vi "Separator_Single_Frame_Displ-3.vi"(3 "error IN":errorcluster, 4 "[IN] Dot matrix with \nstatuses for potentially \nmoving dots":i16[][](array[numeric]), 5 "[IN] Possibly\nMoving (X,Y)":dbl[][](array[numeric]), 6 "[IN] Single Displ":dbl[][](array[numeric])) -> (0 "error OUT":errorcluster, 1 "[OUT] Dot matrix with \nstatuses for potentially \nmoving dots":i16[][](array[numeric]), 2 "[OUT] Single Displ\nw/t problems":dbl[][](array[numeric]))   [LabVIEW 2017]
panel:
  out "Numeric\nof \"+1\" \nevents":i32
  out "2dots to 1dot":dbl[][](array[numeric])
  out "1dot to 2dots":dbl[][](array[numeric])
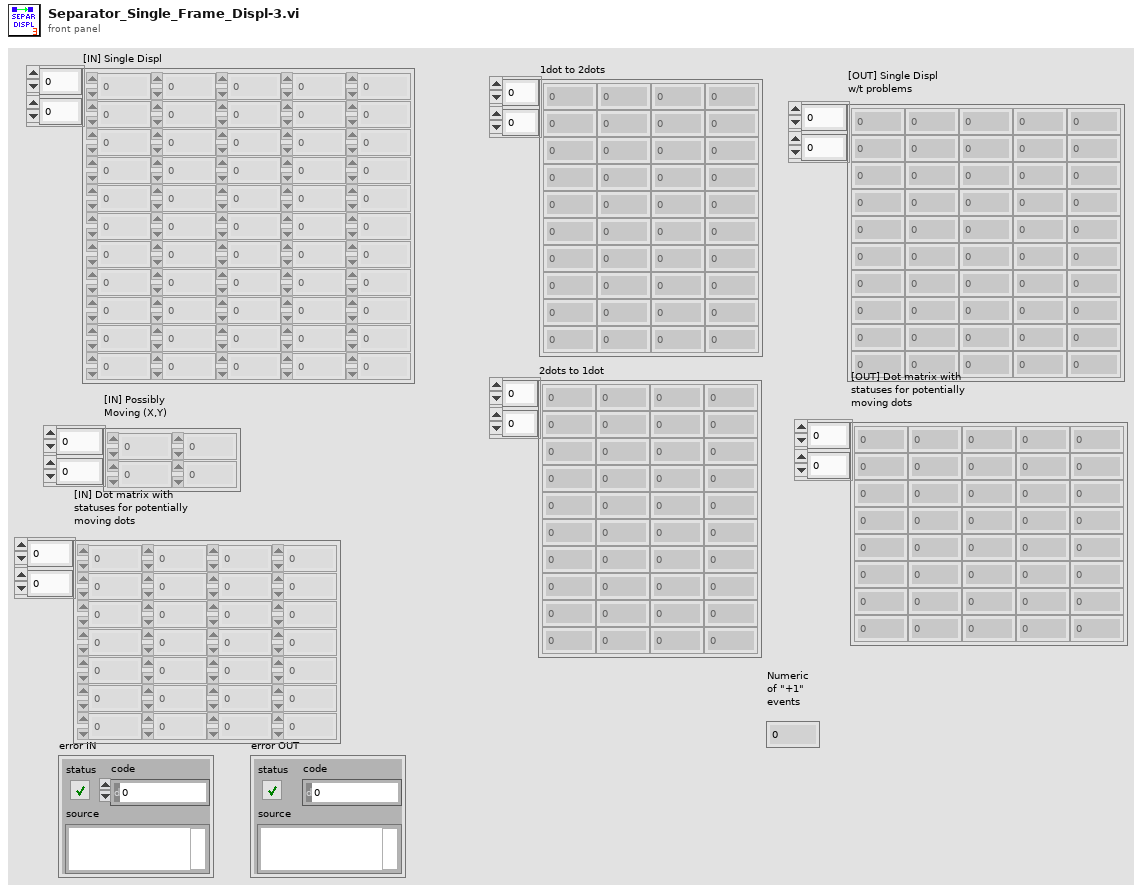
[diagram p1: front panel]
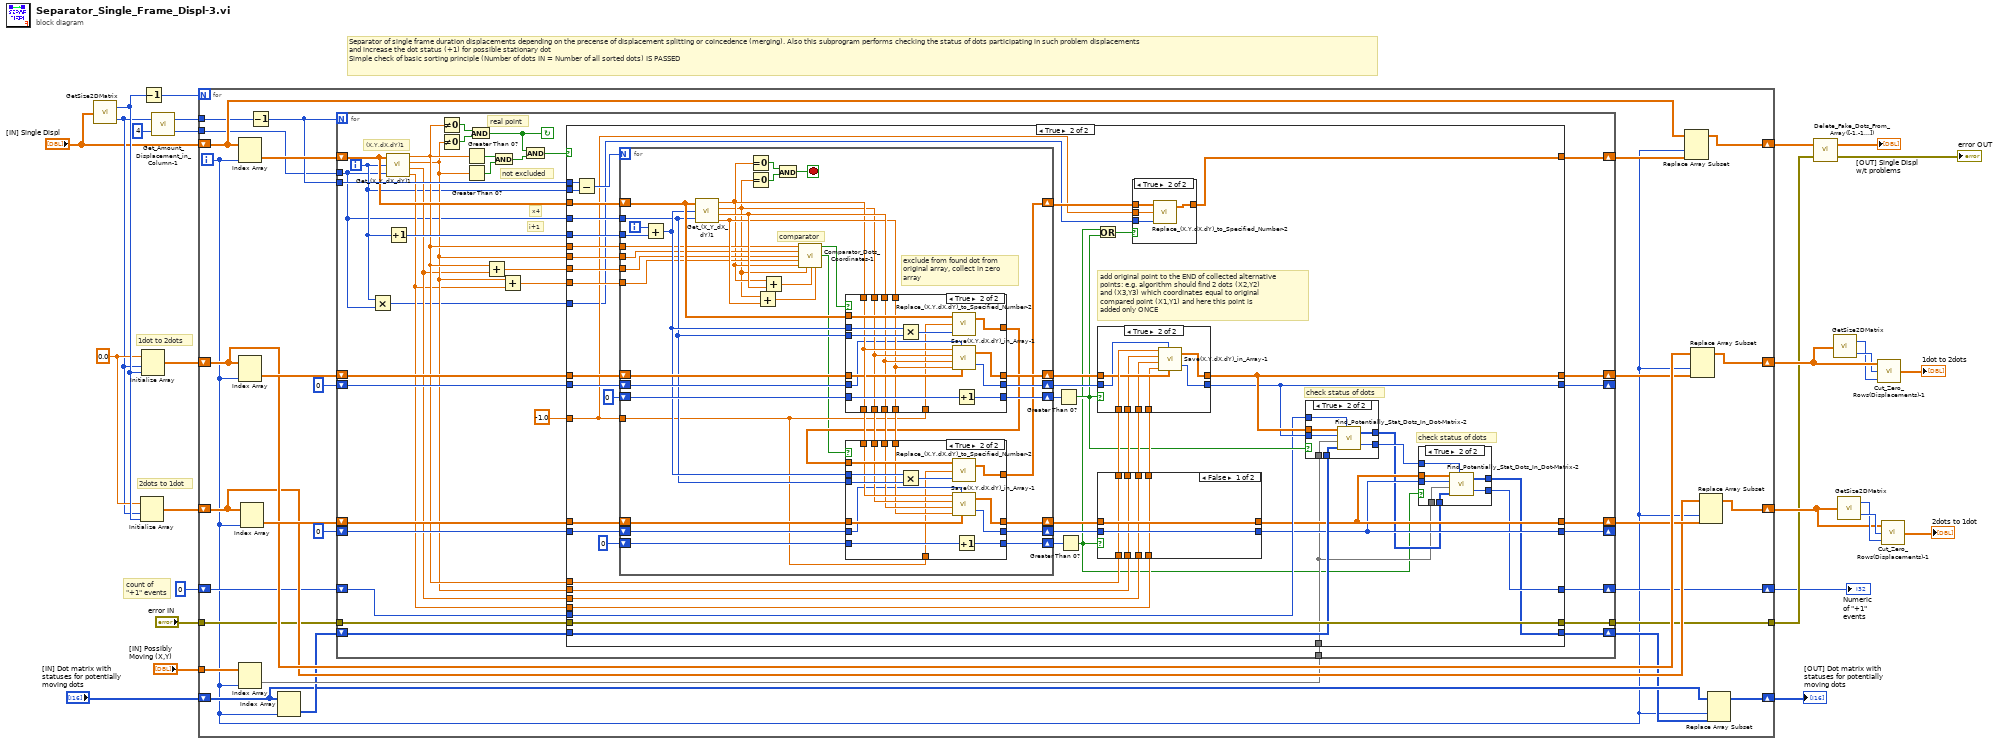
[diagram p0: block diagram]
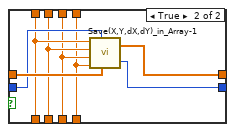
[diagram p6: hidden frame]
diagram:
  w18 = 0.0 ("element")
  # "count of \n\"+1\" events"
  # "2dots to 1dot"
  # "1dot to 2dots"
  # "Separator of single frame duration displacements depending on the precense of displacement splitting or coincedence (merging). Also this subprogram performs checking the status of dots participating in such problem displacements\nand increase the dot status (+1) for possible stationary dot \nSimple check of basic sorting principle (Number of dots IN = Number of all sorted dots) IS PASSED"
  n1 = call "GetSize2DMatrix.vi"("Array IN (2D)"="[IN] Single Displ") -> ("# Cols"=w19:i32, "# Rows"=w13:i32)
  n2 = Initialize Array(w18, w13, w19) -> (w26:dbl[][])
  n3 = Initialize Array(w18, w13, w19) -> (w27:dbl[][])
  n4 = Decrement(x=w19) -> (x-1=w28:i32)
  n5 = call "Get_Amount_Displacement_in_Column-1.vi"("multiplier"=4 ("y"), "# Rows"=w13) -> ("multiplier out"=w10:i32, "Displ amount"=w11:i32)
  n6 = for {
    N: w28 -> [_]
    shift-right: [w45] -> w25
    shift-left: w27 -> [w47]
    shift-right: [w42] -> w20
    shift-left: w26 -> [w43]
    shift-right: [w48] -> w16
    shift-left: "[IN] Single Displ" -> [w50]
    tunnel: "error IN" -> [w41]
    tunnel: [w40] -> w15
    tunnel: w11 -> [w39]
    tunnel: w10 -> [w38]
    tunnel: "[IN] Possibly\nMoving (X,Y)" -> [w37]
    shift-right: [w29] -> w5
    shift-left: "[IN] Dot matrix with \nstatuses for potentially \nmoving dots" -> [w32]
    shift-right: [w33] -> w6
    shift-left: 0 -> [w34]
    i -> [w30]
    n7 = Index Array(array=w50, index (col)=w30) -> (element=w56:dbl[])  [unwired: 1 in]
    n8 = Index Array(array=w47, index (col)=w30) -> (element=w54:dbl[])  [unwired: 1 in]
    n9 = Index Array(array=w37, index (col)=w30) -> (element=w36:dbl[])  [unwired: 1 in]
    n10 = Index Array(array=w43, index (col)=w30) -> (element=w52:dbl[])  [unwired: 1 in]
    n11 = Decrement(x=w39) -> (x-1=w55:i32)
    n12 = Index Array(array=w32, index (col)=w30) -> (element=w35:i16[])  [unwired: 1 in]
    n13 = for {
      N: w55 -> [_]
      tunnel: w38 -> [w66]
      tunnel: w55 -> [w90]
      shift-right: [w72] -> w46
      shift-left: w54 -> [w85]
      shift-right: [w71] -> _
      shift-left: 0 -> [w84]
      shift-right: [w70] -> w44
      shift-left: w52 -> [w83]
      shift-right: [w69] -> _
      shift-left: 0 -> [w82]
      shift-right: [w68] -> w49
      shift-left: w56 -> [w89]
      tunnel: w41 -> [w65]
      tunnel: [w64] -> w40
      tunnel: w36 -> [w61]
      shift-right: [w57] -> w31
      shift-left: w35 -> [w60]
      shift-right: [w58] -> w33
      shift-left: w34 -> [w59]
      i -> [w67]
      stop <- w79 continue-if-true
      # "x4"
      # "i+1"
      # "not excluded"
      # "real point"
      # "(X,Y,dX,dY)1"
      n14 = Multiply(x=w67, y=w66) -> (x*y=w62:i32)
      n15 = call "Get_(X_Y_dX_dY)1.vi"("(X,Y,dX,dY)"=w89, "index"=w67, "multiplier"=w66) -> ("X"=w76:dbl, "Y"=w75:dbl, "dX"=w74:dbl, "dY"=w73:dbl)
      n16 = Increment(x=w67) -> (x+1=w88:i32)
      n17 = Not Equal To 0?(x=w76) -> (x != 0?=w92:bool)
      n18 = Not Equal To 0?(x=w75) -> (x != 0?=w91:bool)
      n19 = Greater Than 0?(x=w76) -> (x > 0?=w81:bool)
      n20 = Greater Than 0?(x=w75) -> (x > 0?=w80:bool)
      n21 = And(x=w92, y=w91) -> (x .and. y?=w79:bool)
      n22 = Add(x=w76, y=w74) -> (x+y=w87:dbl)
      n23 = And(x=w81, y=w80) -> (x .and. y?=w78:bool)
      n24 = Add(x=w75, y=w73) -> (x+y=w86:dbl)
      n25 = And(x=w79, y=w78) -> (x .and. y?=w77:bool)
      n26 = case shown="True" w77 {
        tunnel: w67 -> [_ w148]
        tunnel: w90 -> [_ w149]
        tunnel: w89 -> [w96 w147]
        tunnel: w66 -> [_ w146]
        tunnel: w88 -> [_ w145]
        tunnel: w76 -> [_ w144]
        tunnel: w75 -> [_ w143]
        tunnel: w87 -> [_ w142]
        tunnel: w86 -> [_ w141]
        tunnel: w85 -> [w100 w140]
        tunnel: w84 -> [w99 w139]
        tunnel: w83 -> [w98 w138]
        tunnel: w82 -> [w97 w137]
        tunnel: w76 -> [_ w126]
        tunnel: w75 -> [_ w125]
        tunnel: w74 -> [_ w124]
        tunnel: w73 -> [_ w123]
        tunnel: [w100 w112] -> w72
        tunnel: [w99 w111] -> w71
        tunnel: [w98 w108] -> w70
        tunnel: [w97 w107] -> w69
        tunnel: [w96 w114] -> w68
        tunnel: w65 -> [w95 w133]
        tunnel: [w95 w133] -> w64
        tunnel: -1.0 ("Replacement \nnumber") -> [_ w116]
        tunnel: w62 -> [_ w115]
        tunnel: w61 -> [_ w104]
        tunnel: w60 -> [w93 w110]
        tunnel: w59 -> [w94 w109]
        tunnel: [w94 w102] -> w58
        tunnel: [w93 w101] -> w57
        frame False {
        }
        frame True {
          # "check status of dots"
          # "check status of dots"
          # "add original point to the END of collected alternative \npoints: e.g. algorithm should find 2 dots (X2,Y2) \nand (X3,Y3) which coordinates equal to original \ncompared point (X1,Y1) and here this point is \nadded only ONCE"
          n27 = Subtract(x=w149, y=w148) -> (x-y=w136:i32)
          n28 = for {
            N: w136 -> [_]
            tunnel: w146 -> [w212]
            tunnel: w145 -> [w234]
            tunnel: w144 -> [w206]
            tunnel: w143 -> [w205]
            tunnel: w142 -> [w204]
            tunnel: w141 -> [w203]
            shift-right: [w216] -> w117
            shift-left: w147 -> [w224]
            shift-right: [w227] -> w132
            shift-left: w140 -> [w228]
            shift-right: [w226] -> w131
            shift-left: w139 -> [w225]
            shift-right: [w209] -> w130
            shift-left: w138 -> [w215]
            shift-right: [w208] -> w129
            shift-left: w137 -> [w214]
            shift-right: [w222] -> w127
            shift-left: 0 -> [w223]
            shift-right: [w210] -> w128
            shift-left: 0 -> [w211]
            tunnel: w116 -> [w207]
            i -> [w235]
            stop <- w231 stop-if-true
            # "comparator"
            # "exclude from found dot from \noriginal array, collect in zero \narray"
            n29 = Add(x=w235, y=w234) -> (x+y=w213:i32)
            n30 = call "Get_(X_Y_dX_dY)1.vi"("(X,Y,dX,dY)"=w224, "index"=w213, "multiplier"=w212) -> ("X"=w202:dbl, "Y"=w201:dbl, "dX"=w230:dbl, "dY"=w229:dbl)
            n31 = Equal To 0?(x=w202) -> (x = 0?=w233:bool)
            n32 = Equal To 0?(x=w201) -> (x = 0?=w232:bool)
            n33 = Add(x=w201, y=w229) -> (x+y=w199:dbl)
            n34 = Add(x=w202, y=w230) -> (x+y=w200:dbl)
            n35 = And(x=w233, y=w232) -> (x .and. y?=w231:bool)
            n36 = call "Comparator_Dots_Coordinates-1.vi"("X1"=w206, "Y1"=w205, "(X+dX)1"=w204, "(Y+dY)1"=w203, "X2"=w202, "Y2"=w201, "(X+dX)2"=w200, "(Y+dY)2"=w199) -> ("X1=X2,Y1=Y2 (1)"=w198:bool, "X1(2)=X2(2),Y1(2)=Y2(2) (2)"=w197:bool)  [unwired: 5 in, 1 out]
            n37 = case shown="True" w198 {
              tunnel: w224 -> [w259 w275]
              tunnel: w213 -> [_ w279]
              tunnel: w212 -> [_ w278]
              tunnel: [w259 w273] -> w217
              tunnel: w202 -> [w263 w272]
              tunnel: w201 -> [w262 w270]
              tunnel: w230 -> [w261 w269]
              tunnel: w229 -> [w260 w268]
              tunnel: [w263 w272] -> w221
              tunnel: [w262 w270] -> w220
              tunnel: [w261 w269] -> w219
              tunnel: [w260 w268] -> w218
              tunnel: [w258 w266] -> w227
              tunnel: w228 -> [w258 w271]
              tunnel: [w257 w265] -> w226
              tunnel: w225 -> [w257 w267]
              tunnel: w223 -> [w256 w277]
              tunnel: [w256 w276] -> w222
              tunnel: w207 -> [_ w264]
              frame False {
              }
              frame True {
                n38 = Multiply(x=w279, y=w278) -> (x*y=w274:i32)
                n39 = call "Replace_(X,Y,dX,dY)_to_Specified_Number-2.vi"("Starting index"=w274, "Replacement \nnumber"=w264, "[IN] Sample \narray"=w275) -> ("[OUT] Processed\narray"=w273:dbl[])  [unwired: 1 out]
                n40 = call "Save(X,Y,dX,dY)_in_Array-1.vi"("[IN] Array for Replacement"=w271, "[IN] Starting Position"=w267, "dY"=w268, "dX"=w269, "Y"=w270, "X"=w272) -> ("[OUT] Finish Position"=w265:i32, "[OUT] Array for Replacement"=w266:dbl[])
                n41 = Increment(x=w277) -> (x+1=w276:i32)
              }
            }
            n42 = case shown="True" w197 {
              tunnel: w217 -> [w239 w251]
              tunnel: w213 -> [_ w255]
              tunnel: w212 -> [_ w254]
              tunnel: [w239 w249] -> w216
              tunnel: w221 -> [_ w248]
              tunnel: w220 -> [_ w246]
              tunnel: w219 -> [_ w245]
              tunnel: w218 -> [_ w244]
              tunnel: [w238 w242] -> w209
              tunnel: w215 -> [w238 w247]
              tunnel: [w237 w241] -> w208
              tunnel: w214 -> [w237 w243]
              tunnel: w211 -> [w236 w253]
              tunnel: [w236 w252] -> w210
              tunnel: w207 -> [_ w240]
              frame False {
              }
              frame True {
                n43 = Multiply(x=w255, y=w254) -> (x*y=w250:i32)
                n44 = call "Replace_(X,Y,dX,dY)_to_Specified_Number-2.vi"("Starting index"=w250, "Replacement \nnumber"=w240, "[IN] Sample \narray"=w251) -> ("[OUT] Processed\narray"=w249:dbl[])  [unwired: 1 out]
                n45 = call "Save(X,Y,dX,dY)_in_Array-1.vi"("[IN] Array for Replacement"=w247, "[IN] Starting Position"=w243, "dY"=w244, "dX"=w245, "Y"=w246, "X"=w248) -> ("[OUT] Finish Position"=w241:i32, "[OUT] Array for Replacement"=w242:dbl[])
                n46 = Increment(x=w253) -> (x+1=w252:i32)
              }
            }
          }
          n47 = Greater Than 0?(x=w127) -> (x > 0?=w113:bool)
          n48 = Greater Than 0?(x=w128) -> (x > 0?=w103:bool)
          n49 = Or(x=w103, y=w113) -> (x .or. y?=w118:bool)
          n50 = case shown="False" w103 {
            tunnel: w130 -> [w178 w186]
            tunnel: w129 -> [w177 w185]
            tunnel: w126 -> [w176 w182]
            tunnel: w125 -> [w175 w181]
            tunnel: w124 -> [w174 w180]
            tunnel: w123 -> [w173 w179]
            tunnel: [w177 w183] -> w107
            tunnel: [w178 w184] -> w108
            tunnel: [w176 w182] -> w122
            tunnel: [w175 w181] -> w121
            tunnel: [w174 w180] -> w120
            tunnel: [w173 w179] -> w119
            frame False {
            }
            frame True {
              n51 = call "Save(X,Y,dX,dY)_in_Array-1.vi"("[IN] Array for Replacement"=w186, "[IN] Starting Position"=w185, "dY"=w179, "dX"=w180, "Y"=w181, "X"=w182) -> ("[OUT] Finish Position"=w183:i32, "[OUT] Array for Replacement"=w184:dbl[])
            }
          }
          n52 = case shown="True" w113 {
            tunnel: w132 -> [w188 w195]
            tunnel: w131 -> [w187 w194]
            tunnel: w122 -> [_ w196]
            tunnel: w121 -> [_ w193]
            tunnel: w120 -> [_ w192]
            tunnel: w119 -> [_ w191]
            tunnel: [w187 w189] -> w111
            tunnel: [w188 w190] -> w112
            frame False {
            }
            frame True {
              n53 = call "Save(X,Y,dX,dY)_in_Array-1.vi"("[IN] Array for Replacement"=w195, "[IN] Starting Position"=w194, "dY"=w191, "dX"=w192, "Y"=w193, "X"=w196) -> ("[OUT] Finish Position"=w189:i32, "[OUT] Array for Replacement"=w190:dbl[])
            }
          }
          n54 = case shown="True" w118 {
            tunnel: w117 -> [w168 w172]
            tunnel: w116 -> [_ w171]
            tunnel: w115 -> [_ w170]
            tunnel: [w168 w169] -> w114
            frame False {
            }
            frame True {
              n55 = call "Replace_(X,Y,dX,dY)_to_Specified_Number-2.vi"("Starting index"=w170, "Replacement \nnumber"=w171, "[IN] Sample \narray"=w172) -> ("[OUT] Processed\narray"=w169:dbl[])  [unwired: 1 out]
            }
          }
          n56 = case shown="True" w113 {
            tunnel: w112 -> [_ w167]
            tunnel: w111 -> [_ w166]
            tunnel: w104 -> [_ w165]
            tunnel: w110 -> [w160 w164]
            tunnel: [w160 w163] -> w105
            tunnel: [w159 w162] -> w106
            tunnel: w109 -> [w159 w161]
            frame False {
            }
            frame True {
              n57 = call "Find_Potentially_Stat_Dots_In_Dot-Matrix-2.vi"("[IN] Collecting array"=w167, "Finish Position\n(Collecting arr)"=w166, "[IN] Possibly \nMoving Dots \n(Column)"=w165, "[IN] Dot matrix"=w164, "Number\nof \"+1\""=w161) -> ("[OUT] Dot matrix"=w163:i16[], "Number of such\nassignments"=w162:i32)
            }
          }
          n58 = case shown="True" w103 {
            tunnel: w108 -> [_ w158]
            tunnel: w107 -> [_ w157]
            tunnel: w104 -> [_ w156]
            tunnel: w105 -> [w151 w155]
            tunnel: [w151 w154] -> w101
            tunnel: [w150 w153] -> w102
            tunnel: w106 -> [w150 w152]
            frame False {
            }
            frame True {
              n59 = call "Find_Potentially_Stat_Dots_In_Dot-Matrix-2.vi"("[IN] Collecting array"=w158, "Finish Position\n(Collecting arr)"=w157, "[IN] Possibly \nMoving Dots \n(Column)"=w156, "[IN] Dot matrix"=w155, "Number\nof \"+1\""=w152) -> ("[OUT] Dot matrix"=w154:i16[], "Number of such\nassignments"=w153:i32)
            }
          }
        }
      }
    }
    n60 = Replace Array Subset(array=w50, new element=w49, index (col)=w30) -> (w48:dbl[][])  [unwired: 1 in]
    n61 = Replace Array Subset(array=w47, new element=w46, index (col)=w30) -> (w45:dbl[][])  [unwired: 1 in]
    n62 = Replace Array Subset(array=w43, new element=w44, index (col)=w30) -> (w42:dbl[][])  [unwired: 1 in]
    n63 = Replace Array Subset(array=w32, new element=w31, index (col)=w30) -> (w29:i16[][])  [unwired: 1 in]
  }
  "Numeric\nof \"+1\" \nevents" <- w6
  "[OUT] Dot matrix with \nstatuses for potentially \nmoving dots" <- w5
  n64 = call "Delete_Fake_Dots_From_Array([-1,-1...]).vi"("error IN"=w15, "[IN] Source Array"=w16) -> ("error OUT"=→"error OUT":errorcluster, "[OUT] Filtered Array (X,Y,dX,dY)"=→"[OUT] Single Displ\nw/t problems":dbl[][])
  n65 = call "GetSize2DMatrix.vi"("Array IN (2D)"=w25) -> ("# Cols"=w23:i32, "# Rows"=w24:i32)
  n66 = call "GetSize2DMatrix.vi"("Array IN (2D)"=w20) -> ("# Cols"=w21:i32, "# Rows"=w22:i32)
  n67 = call "Cut_Zero_Rows(Displacements)-1.vi"("# Cols"=w23, "# Rows"=w24, "Array IN"=w25) -> ("Array OUT"=→"1dot to 2dots":dbl[][])
  n68 = call "Cut_Zero_Rows(Displacements)-1.vi"("# Cols"=w21, "# Rows"=w22, "Array IN"=w20) -> ("Array OUT"=→"2dots to 1dot":dbl[][])
